vi "Set ICP1-DO Changed bit.vi"(7 "Wait (F)":bool, 8 "error in (no error)":errorcluster, 9 "Value":bool, 10 "DO Channel":T1, 11 "IO in":refnum<class "IO.lvclass">) -> (0 "error out":errorcluster, 3 "IO out":refnum<class "IO.lvclass">)   [LabVIEW 2022 SP3, in "IO.lvclass"]
uses:
  IO.lvclass
  Typedefs/ICP1-D0 Channel Names.ctl
  Typedefs/API Command Cluster.ctl
  Typedefs/API Command Enum.ctl
  Typedefs/DO Value API Data.ctl
  Typedefs/Device Names.ctl
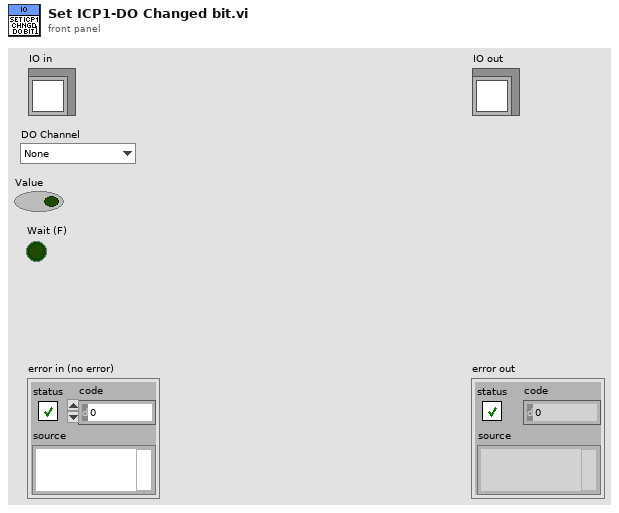
[diagram p1: front panel]
types:
  T1 = typedef "IO.lvclass/ICP1-D0 Channel Names.ctl" = enum16{"None", "Meniscus Pressure Reg PWR - R1", "Meniscus Pressure Reg PWR - R2", "Meniscus Pressure Reg PWR - R3", "Meniscus Pressure Reg PWR - R4", "Meniscus Pressure Reg PWR - R5", "Meniscus Pressure Reg PWR - R6", "Clear Stage Alarm", "Servo ON", "Purge Valve Open - R1", "Purge Valve Open - R2", "Purge Valve Open - R3", "Purge Valve Open - R4", "Purge Valve Open - R5", "Purge Valve Open - R6"}
  T2 = typedef "IO.lvclass/Device Names.ctl" = enum16{"ICP1-DO", "ICP2-DI", "ICP2-DO", "ICP1-AI", "ICP1-AO", "ICP2-AO"}
  T3 = typedef "IO.lvclass/DO Value API Data.ctl" = cluster{"Device Name":T2, "Value":bool, "Index":i32}
  T4 = typedef "IO.lvclass/API Command Enum.ctl" = enum16{"Set DO Value", "Set AO Value", "Purge PH"}
  T5 = typedef "IO.lvclass/API Command Cluster.ctl" = cluster{"Command":T4, "Arguments":string, "Data":variant}
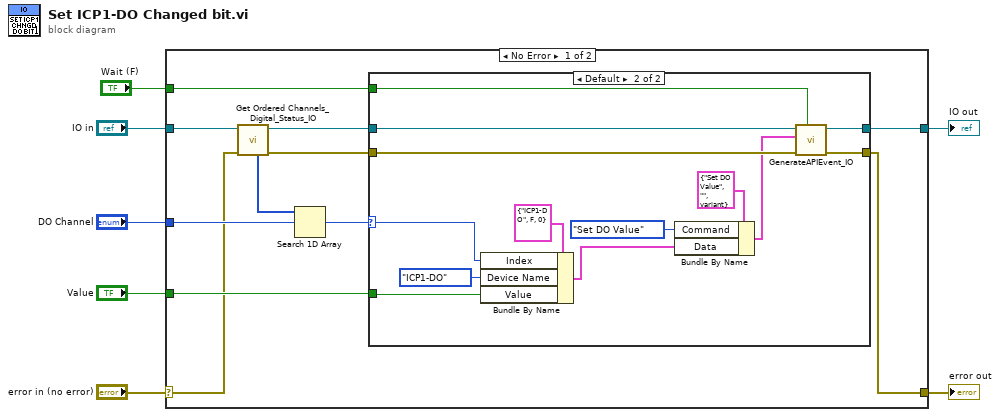
[diagram p0: block diagram]
diagram:
  n1 = case shown="No Error" "error in (no error)" {
    selector: "error in (no error)" -> [w12 w35]
    tunnel: [w11 w35] -> w6
    tunnel: [w15 w34] -> w4
    tunnel: "IO in" -> [w18 w34]
    tunnel: "DO Channel" -> [w17 _]
    tunnel: "Value" -> [w14 _]
    tunnel: "Wait (F)" -> [w8 _]
    frame No Error {
      n2 = call-dynamic "Get Ordered Channels_Digital_Status_IO.vi"("error in (no error)"=w12, "IO in"=w18) -> ("error out"=w13:errorcluster, "IO out"=w16:refnum<class "IO.lvclass">, "Ordered ICP1-DO Channels"=w9:T1[])  [unwired: 5 in, 2 out]
      n3 = Search 1D Array(1D array=w9, element=w17) -> (index of element=w10:i32)  [unwired: 1 in]
      n4 = case shown="Default" w10 {
        selector: w10 -> [_ w25]
        tunnel: w16 -> [w20 w21]
        tunnel: [w20 w32] -> w15
        tunnel: w14 -> [_ w26]
        tunnel: w13 -> [w19 w33]
        tunnel: [w19 w31] -> w11
        tunnel: w8 -> [_ w22]
        frame -1 {
        }
        frame Default {
          n5 = Bundle By Name(cluster=T3 {"Device Name"=enum."ICP1-DO", "Value"=FALSE, "Index"=0} ("DO Value Input"), "Index"=w25, "Device Name"=Device_Names."ICP1-DO", "Value"=w26) -> (w24:T3)
          n6 = Bundle By Name(cluster=T5 {"Command"=enum."Set DO Value", "Arguments"="", "Data"=variant} ("API Command Cluster"), "Command"=API_Command_Enum."Set DO Value", "Data"=w24) -> (w28:T5)
          n7 = call "GenerateAPIEvent_IO.vi"("Wait (F)"=w22, "error in (no error)"=w33, "API Command Cluster"=w28, "IO.lvclass"=w21) -> ("error out"=w31:errorcluster, "IO.lvclass out"=w32:refnum<class "IO.lvclass">)  [unwired: 6 in]
        }
      }
    }
    frame Error {
    }
  }
  "error out" <- w6
  "IO out" <- w4
